vi "send_switch_counter_to_AnalysisObj.vi"(0 "SessionID":string, 5 "switch name":string, 7 "counter value":dbl, 11 "error in (no error)":errorcluster) -> (15 "error out":errorcluster)   [LabVIEW 2018]
doc: "sendds the data to the AnalysisSession (SessionID) and stores them in the AnalysisDataArray"
uses:
  Classes/Analysis/Analysis.lvclass
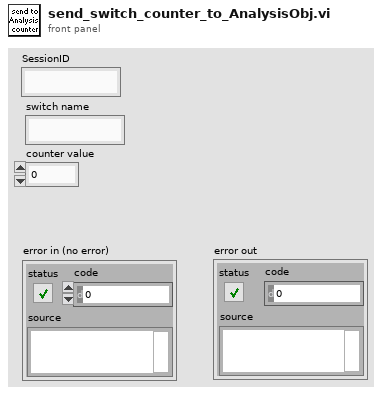
[diagram p1: front panel]
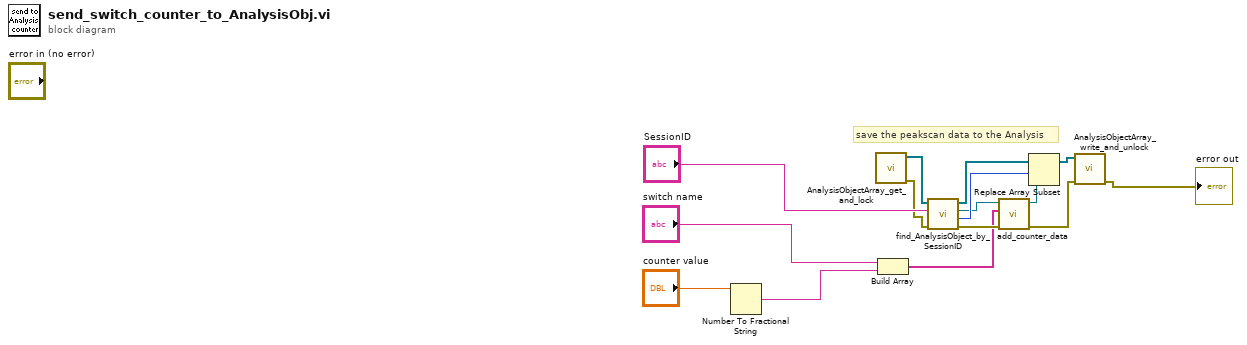
[diagram p0: block diagram]
diagram:
  # "save the peakscan data to the Analysis"
  n1 = Number To Fractional String(number="counter value") -> (F-format string=w14:string)  [unwired: 3 in]
  n2 = call "AnalysisObjectArray_get_and_lock.vi"() -> ("error out"=w5:errorcluster, "AnalysisObjects"=w2:refnum<class "Analysis.lvclass">[])  [unwired: 10 in]
  n3 = Build Array("switch name", w14) -> (w1:string[])
  n4 = call "find_AnalysisObject_by_SessionID.vi"("error in (no error)"=w5, "SessionID"="SessionID", "AnalysisObjects in"=w2) -> ("error out"=w4:errorcluster, "index of found"=w8:i32, "found AnalyisObject"=w3:refnum<class "Analysis.lvclass">, "AnalysisObjects out"=w6:refnum<class "Analysis.lvclass">[])  [unwired: 5 in]
  n5 = call-dynamic "add_counter_data.vi"("error in (no error)"=w4, "counter data"=w1, "Analysis in"=w3) -> ("error out"=w10:errorcluster, "Analysis out"=w7:refnum<class "Analysis.lvclass">)  [unwired: 7 in]
  n6 = Replace Array Subset(array=w6, new element=w7, index=w8) -> (w9:refnum<class "Analysis.lvclass">[])
  n7 = call "AnalysisObjectArray_write_and_unlock.vi"("error in (no error)"=w10, "AnalysisObjects"=w9) -> ("error out"=→"error out":errorcluster)  [unwired: 9 in]
